vi "ExtendedFloat (Scalar) to String.vi"(7 "Use System Default Notation (F)":bool, 11 "Value (Extended)":ext format="%#_34g") -> (3 "Value (String)":string)   [LabVIEW 2013, in "OpenScalar.lvlib"]
uses:
  OpenScalar.lvlib
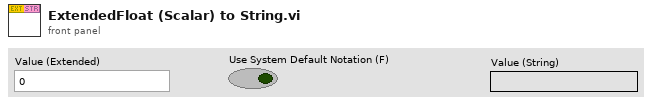
[diagram p1: front panel]
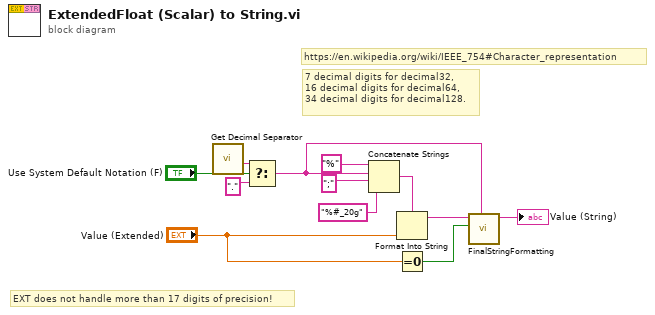
[diagram p0: block diagram]
diagram:
  # "EXT does not handle more than 17 digits of precision!"
  # "7 decimal digits for decimal32,\n16 decimal digits for decimal64,\n34 decimal digits for decimal128."
  # "https://en.wikipedia.org/wiki/IEEE_754#Character_representation"
  n1 = call "Get Decimal Separator.vi"() -> ("System Decimal separator"=w12:string)  [unwired: 11 in]
  n2 = Select(t=w12, s="Use System Default Notation (F)", f="." ("format string")) -> (s? t:f=w3:string)
  n3 = Concatenate Strings("%" ("format string"), w3, ";" ("regular expression"), "%#_20g" ("format string")) -> (w7:string)
  n4 = Format Into String(format string=w7, "Value (Extended)") -> (resulting string=w4:string)  [unwired: 2 in, 1 out]
  n5 = Equal To 0?(x="Value (Extended)") -> (x = 0?=w2:bool)
  n6 = call "FinalStringFormatting.vi"("Decimal Notation (.)"=w3, "Equals Zero?"=w2, "String in"=w4) -> ("String out"=→"Value (String)":string)  [unwired: 8 in]
